vi "In_S2F35.vi"(8 "error in (no error)":errorcluster, 11 "S2 Message Class in":refnum<class "S2 Message Class.lvclass">) -> (0 "error out":errorcluster, 1 "OK?":bool, 2 "S2F35":T1, 3 "S2 Message Class out":refnum<class "S2 Message Class.lvclass">)   [LabVIEW 2020, in "SECS Communication.lvlib" / "S2 Message Class.lvclass"]
uses:
  S2 Message Class.lvclass
  D:/Dropbox/SECS/SECS_GEM v1.0.7/Com/SECS Communication/SECS-II Class/SECS-II Class.lvclass
  S2F35.ctl
  SECS-II Class/SECS-II Class.lvclass/SECS-II Class.ctl
  SECS-II Class/Variant To Data_U4.vi
  SECS-II Class/SECS-II Class.lvclass
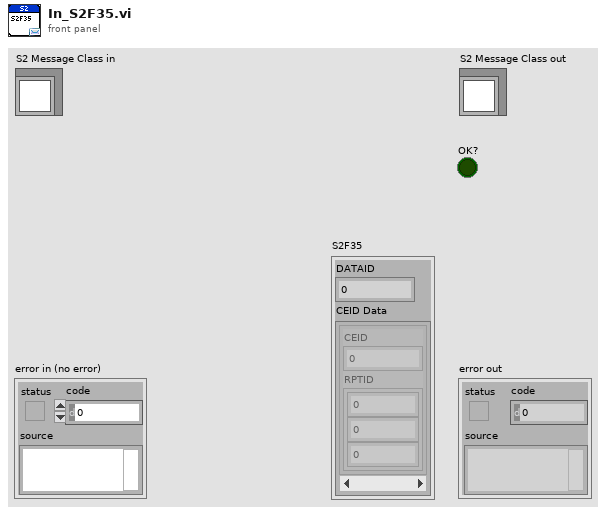
[diagram p1: front panel]
types:
  T1 = typedef "SECS Communication.lvlib/S2 Message Class.lvclass/S2F35.ctl" = cluster{"DATAID":u32, "CEID Data":cluster{"CEID":u32, "RPTID":u32[]}[]}
  T2 = typedef "SECS Communication.lvlib/SECS-II Class.lvclass/Message Data.ctl" = cluster{"Index":i32, "Data Item Format":T3, "Format Code":T4, "Parent Index":i32, "Child Index":i32[], "Data":variant}
  T3 = typedef "SECS Communication.lvlib/SECS-II Class.lvclass/Data Item Format.ctl" = enum16{"Data Type", "Value"}
  T4 = typedef "SECS Communication.lvlib/SECS-II Class.lvclass/Format Code.ctl" = enum16{"L", "A", "B", "Boolean", "J", "I1", "I2", "I4", "I8", "U1", "U2", "U4", "U8", "F4", "F8", "Char"}
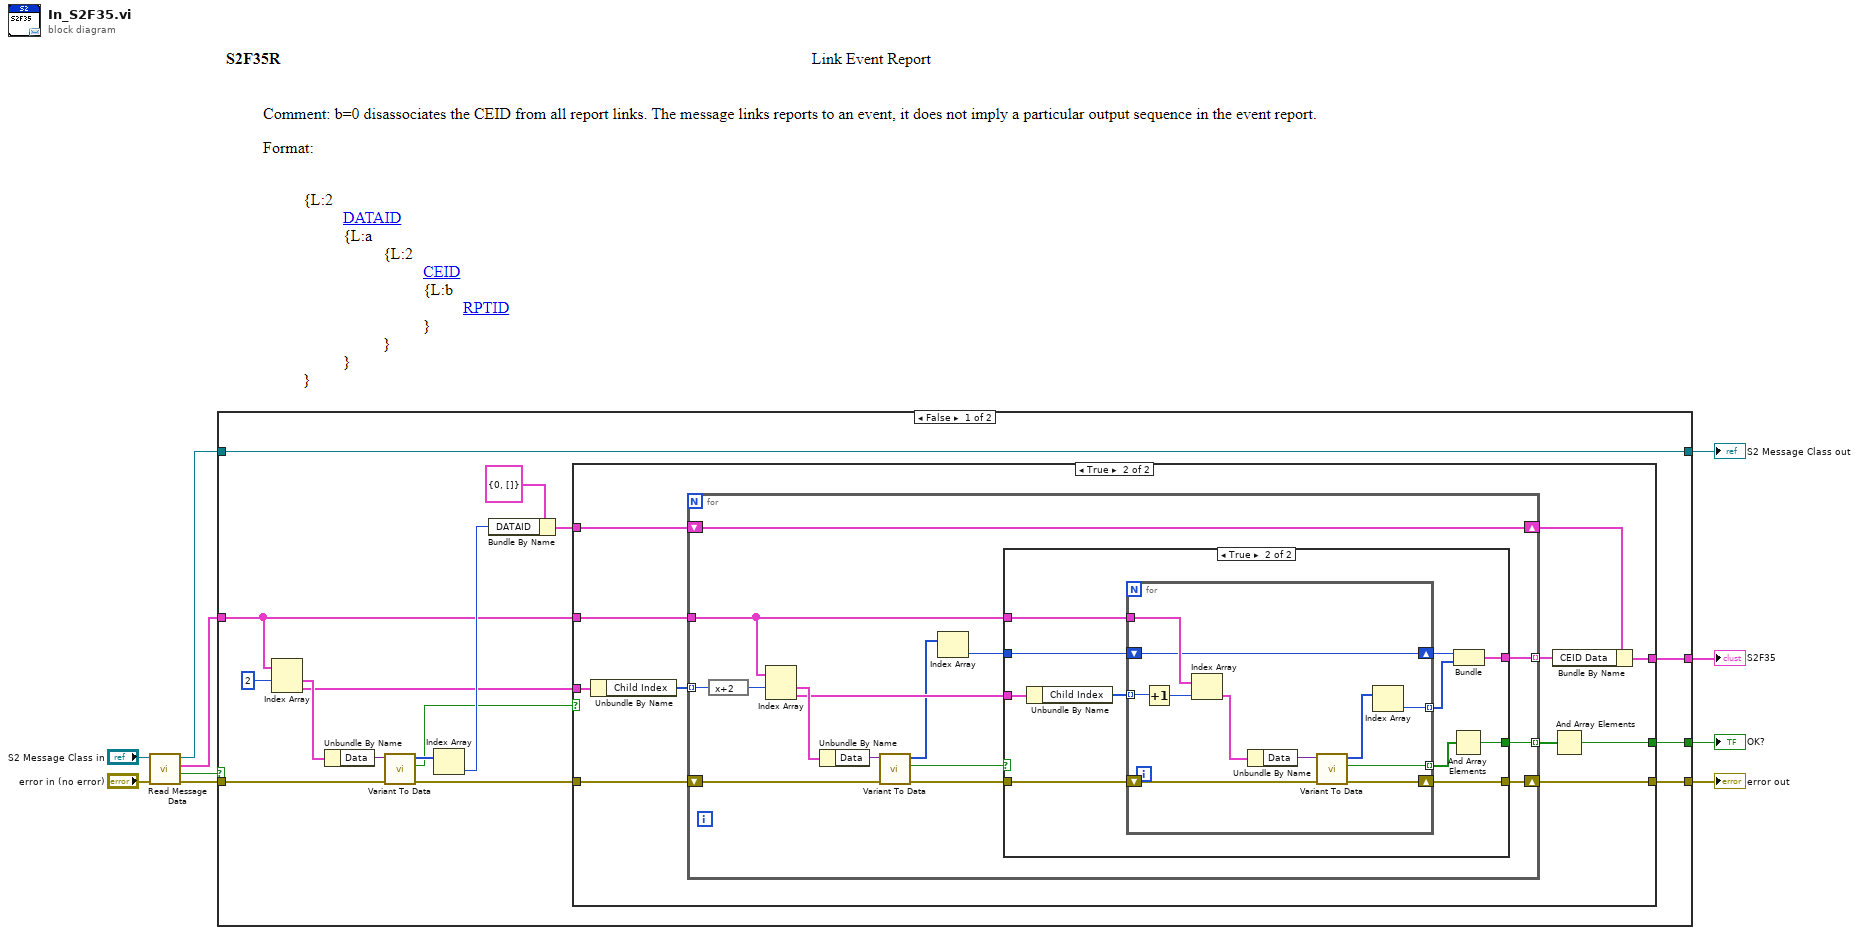
[diagram p0: block diagram]
diagram:
  n1 = call "Read Message Data.vi"("error in (no error)"="error in (no error)", "SECS-II Class in"="S2 Message Class in") -> ("error out"=w10:errorcluster, "Empty?"=w9:bool, "Message Data"=w7:T2[], "SECS-II Class out"=w8:refnum<class "S2 Message Class.lvclass">)  [unwired: 6 in]
  n2 = case shown="False" w9 {
    tunnel: w10 -> [w24 w77]
    tunnel: w8 -> [w15 w78]
    tunnel: w7 -> [w16 _]
    tunnel: [w15 w78] -> w5
    tunnel: [w14 w77] -> w6
    tunnel: [w13 _] -> w4
    tunnel: [w12 _] -> w3
    frame False {
      n3 = Index Array(array=w16, index #1=2 ("index")) -> (element #1=w25:T2, element #2=w17:T2)  [unwired: 1 in]
      n4 = Unbundle By Name(w25) -> ("Data"=w23:variant)
      n5 = call-poly "Variant To Data.vi"("error in (no error)"=w24, "Variant"=w23) -> ("error out"=w20:errorcluster, "OK?"=w19:bool, "Data"=w22:u32[])  [unwired: 7 in]
      n6 = Index Array(array=w22) -> (element=w21:u32)  [unwired: 1 in]
      n7 = Bundle By Name(cluster=T1 {"DATAID"=0, "CEID Data"=[]} ("S2F35"), "DATAID"=w21) -> (w18:T1)
      n8 = case shown="True" w19 {
        tunnel: w20 -> [w27 w36]
        tunnel: w18 -> [_ w32]
        tunnel: w17 -> [_ w38]
        tunnel: w16 -> [_ w35]
        tunnel: [w27 w30] -> w14
        tunnel: [_ w29] -> w13
        tunnel: [_ w28] -> w12
        frame False {
        }
        frame True {
          n9 = Unbundle By Name(w38) -> ("Child Index"=w37:i32[])
          n10 = for {
            tunnel: w37 -> [w40] mode=indexing
            shift-right: [w43] -> w30
            shift-left: w36 -> [w52]
            tunnel: w35 -> [w47]
            tunnel: [w44] -> w34 mode=indexing
            tunnel: [w42] -> w33 mode=indexing
            shift-right: [w41] -> w31
            shift-left: w32 -> [w41]
            n11 = expression code="x+2"(w40) -> (w39:i32)
            n12 = Index Array(array=w47, index #1=w39) -> (element #1=w51:T2, element #2=w48:T2)  [unwired: 1 in]
            n13 = Unbundle By Name(w51) -> ("Data"=w53:variant)
            n14 = call-poly "Variant To Data.vi"("error in (no error)"=w52, "Variant"=w53) -> ("error out"=w50:errorcluster, "OK?"=w49:bool, "Data"=w46:u32[])  [unwired: 7 in]
            n15 = Index Array(array=w46) -> (element=w45:u32)  [unwired: 1 in]
            n16 = case shown="True" w49 {
              tunnel: w50 -> [w54 w64]
              tunnel: w48 -> [_ w65]
              tunnel: w47 -> [_ w62]
              tunnel: w45 -> [_ w61]
              tunnel: [_ w57] -> w44
              tunnel: [_ w56] -> w42
              tunnel: [w54 w55] -> w43
              frame False {
              }
              frame True {
                n17 = Unbundle By Name(w65) -> ("Child Index"=w63:i32[])
                n18 = for {
                  shift-right: [w69] -> w55
                  shift-left: w64 -> [w70]
                  tunnel: w63 -> [w76] mode=indexing
                  tunnel: w62 -> [w75]
                  shift-right: [w71] -> w60
                  shift-left: w61 -> [w71]
                  tunnel: [w68] -> w58 mode=indexing
                  tunnel: [w66] -> w59 mode=indexing
                  n19 = Increment(x=w76) -> (x+1=w74:i32)
                  n20 = Index Array(array=w75, index=w74) -> (element=w73:T2)
                  n21 = Unbundle By Name(w73) -> ("Data"=w72:variant)
                  n22 = call-poly "Variant To Data.vi"("error in (no error)"=w70, "Variant"=w72) -> ("error out"=w69:errorcluster, "OK?"=w68:bool, "Data"=w67:u32[])  [unwired: 7 in]
                  n23 = Index Array(array=w67) -> (element=w66:u32)  [unwired: 1 in]
                }
                n24 = And Array Elements(Boolean array=w58) -> (logical AND=w57:bool)
                n25 = Bundle("Data"=w60, w59) -> (w56:cluster{"Data":u32, u32[]})  [unwired: 1 in]
              }
            }
          }
          n26 = Bundle By Name(cluster=w31, "CEID Data"=w33) -> (w29:T1)
          n27 = And Array Elements(Boolean array=w34) -> (logical AND=w28:bool)
        }
      }
    }
    frame True {
    }
  }
  "error out" <- w6
  "S2 Message Class out" <- w5
  "S2F35" <- w4
  "OK?" <- w3
